vi "run.vi"(8 "error in (no error)":errorcluster, 11 "Protocol_Generic in":refnum<class "Protocol_Generic.lvclass">) -> (0 "error out":errorcluster, 3 "Protocol_Generic out":refnum<class "Protocol_Generic.lvclass">)   [LabVIEW 2011, in "Protocol_Generic.lvclass"]
uses:
  Protocol_Generic.lvclass
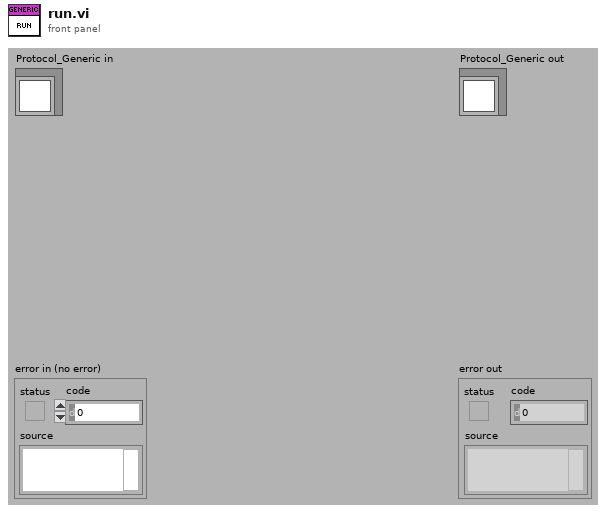
[diagram p1: front panel]
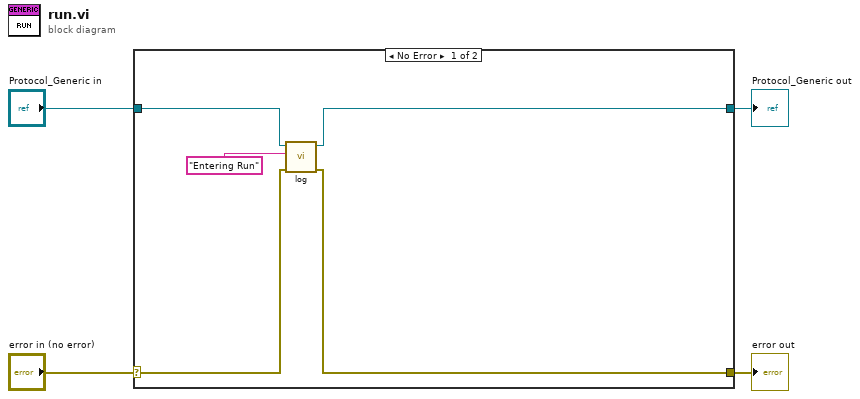
[diagram p0: block diagram]
diagram:
  n1 = case shown="No Error" "error in (no error)" {
    selector: "error in (no error)" -> [w7 w11]
    tunnel: [w6 w11] -> w3
    tunnel: [w5 w10] -> w1
    tunnel: "Protocol_Generic in" -> [w8 w10]
    frame No Error {
      n2 = call-dynamic "log.vi"("error in (no error)"=w7, "logLineIn"="Entering Run", "Protocol_Generic in"=w8) -> ("error out"=w6:errorcluster, "Protocol_Generic out"=w5:refnum<class "Protocol_Generic.lvclass">)  [unwired: 7 in]
    }
    frame Error {
    }
  }
  "error out" <- w3
  "Protocol_Generic out" <- w1
